vi "Write Test Parameters.vi"(10 "Test Parameters":T1 {"Cycle profile"."Pause After" min=1.0 max=600.0 format="%.1f"; "Cycle profile"."Force Setpoint" min=-556.0 max=556.0 format="%.1f"; "Number of cycles for complete test" min=1}, 11 "StartAutomatedTest in":refnum<class "StartAutomatedTest.lvclass">) -> (3 "StartAutomatedTest out":refnum<class "StartAutomatedTest.lvclass">)   [LabVIEW 2013, in "StartAutomatedTest.lvclass"]
uses:
  StartAutomatedTest.lvclass
  Configuration/Test Parameters.ctl
  Configuration/CycleProfileConfig.ctl
  StartAutomatedTest.lvclass/StartAutomatedTest.ctl
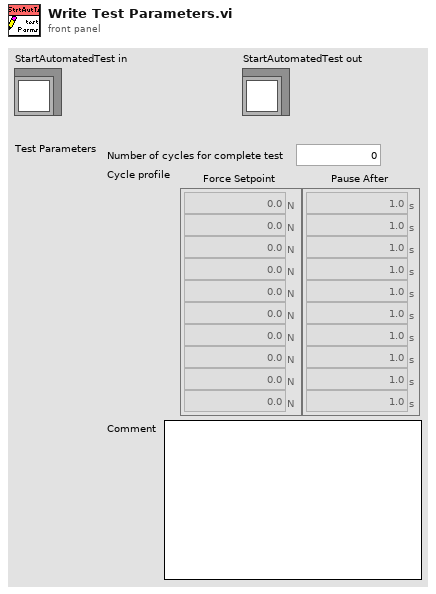
[diagram p1: front panel]
types:
  T1 = typedef "Test Parameters.ctl" = cluster{"Number of cycles for complete test":u32, "Cycle profile":T2, "Comment":string}
  T2 = typedef "CycleProfileConfig.ctl" = cluster{"Force Setpoint":dbl[unit][], "Pause After":dbl[unit][]}
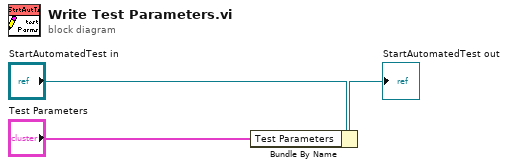
[diagram p0: block diagram]
diagram:
  n1 = Bundle By Name(cluster="StartAutomatedTest in", "Test Parameters"="Test Parameters") -> (→"StartAutomatedTest out":refnum<class "StartAutomatedTest.lvclass">)
